vi "MGI Get Cluster Index.vi"(8 "Error In":errorcluster, 9 "Mode":T1(ring), 10 "Name":string, 11 "Cluster In":variant) -> (0 "Error Out":errorcluster, 2 "Index":i32)   [LabVIEW 2020]
doc: "This VI returns the tabbing order index of the element or subelement in <b>Cluster In</b> named <b>Name</b>. A -1 is returned if the element is not found. What <b>Index</b> means depends on <b>Mode</b>:\n\nInclude all elements and subelements: recurses all clusters and subclusters and increments for each cluster or any other data type. <b>Index</b> returns the element's order among all elements, no matter the level.\n\nFirst level only: only looks at the elements of <b>Cluster In</b>. Will not recurse on any subclusters of <b>Cluster In</b>. In this case, <b>Index</b> refers to the tabbing order of <b>Cluster In</b>.\n\nIndex in lowest level: once an element with <b>Name</b> is found, its tab order index in its owning cluster is returned in <b>Index</b>.\n\nAuthored by Robert C. Mortensen\nsupport@mooregoodideas.com\nwww.mooregoodideas.com\n\nCopyright (c) 2010, Moore Good Ideas, Inc.\n\nAll rights reserved.\n\nRedistribution and use in source and binary forms, with or without modification, are permitted provided that the following conditions are met:\n\n * Redistributions of source code must retain the above copyright notice, this list of conditions and the following disclaimer.\n * Redistributions in binary form must reproduce the above copyright notice, this list of conditions and the following disclaimer in the documentation and/or other materials provided with the distribution.\n * Neither the name of Moore Good Ideas, Inc. nor the names of its contributors may be used to endorse or promote products derived from this software without specific prior written permission.\n\nTHIS SOFTWARE IS PROVIDED BY THE COPYRIGHT HOLDERS AND CONTRIBUTORS \"AS IS\" AND ANY EXPRESS OR IMPLIED WARRANTIES, INCLUDING, BUT NOT LIMITED TO, THE IMPLIED WARRANTIES OF MERCHANTABILITY AND FITNESS FOR A PARTICULAR PURPOSE ARE DISCLAIMED. IN NO EVENT SHALL THE COPYRIGHT OWNER OR CONTRIBUTORS BE LIABLE FOR ANY DIRECT, INDIRECT, INCIDENTAL, SPECIAL, EXEMPLARY, OR CONSEQUENTIAL DAMAGES (INCLUDING, BUT NOT LIMITED TO, PROCUREMENT OF SUBSTITUTE GOODS OR SERVICES; LOSS OF USE, DATA, OR PROFITS; OR BUSINESS INTERRUPTION) HOWEVER CAUSED AND ON ANY THEORY OF LIABILITY, WHETHER IN CONTRACT, STRICT LIABILITY, OR TORT (INCLUDING NEGLIGENCE OR OTHERWISE) ARISING IN ANY WAY OUT OF THE USE OF THIS SOFTWARE, EVEN IF ADVISED OF THE POSSIBILITY OF SUCH DAMAGE."
uses:
  <vilib>/Utility/VariantDataType/VariantType.lvlib
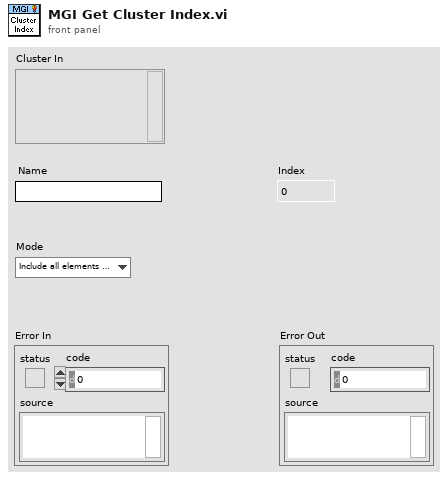
[diagram p1: front panel]
types:
  T1 = enum16{"Include all elements and subelements", "First level only", "Index in lowest level"}
  T2 = typedef "VariantType.lvlib/Type.ctl" = enum8{"Invalid Type", "Void", "I8", "I16", "I32", "I64", "U8", "U16", "U32", "U64", "Single Float", "Double Float", "Extended Float", "Single Complex", "Double Complex", "Extended Complex", "Enum U8", "Enum U16", "Enum U32", "Enum U64", "Single Float With Unit", "Double Float With Unit", "Extended Float With Unit", "Single Complex with Unit", "Double Complex with Unit", "Extended Complex with Unit", "Boolean", "String", "Path", "Picture", "Tag", "Array", "Cluster", "Variant", "LV Variant", "Waveform", "Timestamp", "Digital Waveform", "Digital Data", "ExpressData", "Refnum", "External Data", "VI", "Poly VI", "LabVIEW Class Instance", "Fixed Point"}
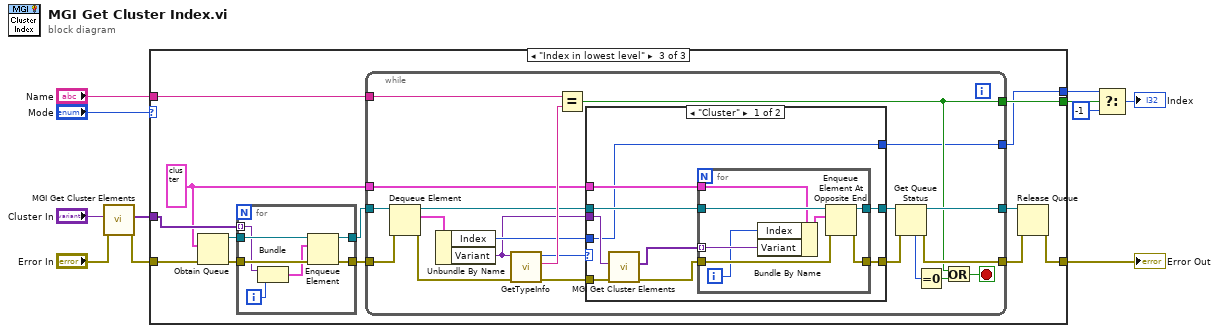
[diagram p0: block diagram]
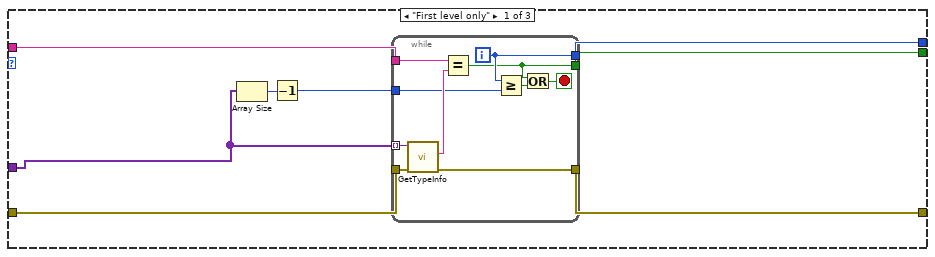
[diagram p2: hidden frame]
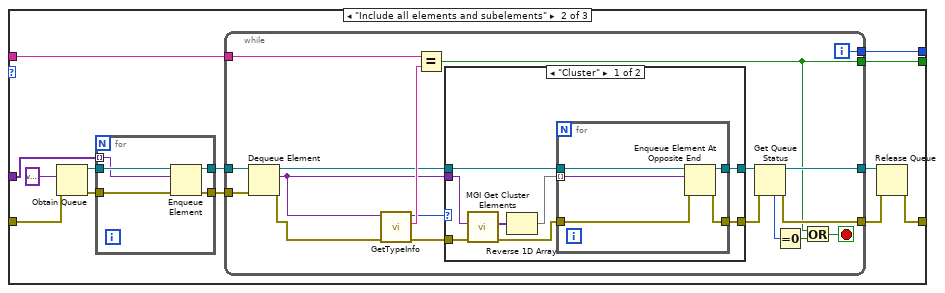
[diagram p3: hidden frame]
diagram:
  n1 = call <userlib>:"MGI Get Cluster Elements.vi"("Error In"="Error In", "Cluster"="Cluster In") -> ("Error Out"=w9:errorcluster, "Cluster Elements"=w8:variant[])  [unwired: 8 in]
  n2 = case shown="\"Index in lowest level\"" "Mode" {
    tunnel: w9 -> [w16 w42 w93]
    tunnel: w8 -> [w14 w39 w90]
    tunnel: "Name" -> [w19 w35 w87]
    tunnel: [w15 w32 w84] -> w6
    tunnel: [w18 w31 w82] -> w5
    tunnel: [w17 w30 w83] -> w2
    frame "First level only" {
      n3 = Array Size(array=w14) -> (size(s)=w13:i32)
      n4 = Decrement(x=w13) -> (x-1=w12:i32)
      n5 = while {
        tunnel: w19 -> [w28]
        tunnel: [w25] -> w15
        tunnel: [w23] -> w18
        tunnel: [w21] -> w17
        tunnel: w14 -> [w27] mode=indexing
        tunnel: w16 -> [w26]
        tunnel: w12 -> [w22]
        i -> [w23]
        stop <- w24 stop-if-true
        n6 = call <vilib>:"GetTypeInfo.vi"("error in (no error)"=w26, "Variant"=w27) -> ("error out"=w25:errorcluster, "Name"=w29:string)  [unwired: 5 in, 3 out]
        n7 = Equal?(x=w28, y=w29) -> (x = y?=w21:bool)
        n8 = Greater Or Equal?(x=w23, y=w22) -> (x >= y?=w20:bool)
        n9 = Or(x=w21, y=w20) -> (x .or. y?=w24:bool)
      }
    }
    frame "Include all elements and subelements" {
      n10 = Obtain Queue(element data type=variant, error in (no error)=w42) -> (queue out=w40:refnum<queue>, error out=w41:errorcluster)  [unwired: 3 in, 1 out]
      n11 = for {
        tunnel: w41 -> [w80]
        tunnel: w40 -> [w79]
        tunnel: w39 -> [w78] mode=indexing
        tunnel: [w77] -> w36
        tunnel: [w76] -> w37
        n12 = Enqueue Element(queue=w79, element=w78, error in (no error)=w80) -> (queue out=w76:refnum<queue>, error out=w77:errorcluster)  [unwired: 1 in, 1 out]
      }
      n13 = while {
        tunnel: w37 -> [w59]
        tunnel: w36 -> [w60]
        tunnel: w35 -> [w53]
        tunnel: [w46] -> w34
        tunnel: [w45] -> w33
        tunnel: [w44] -> w31
        tunnel: [w43] -> w30
        i -> [w44]
        stop <- w56 stop-if-true
        n14 = Dequeue Element(queue=w59, error in (no error)=w60) -> (queue out=w51:refnum<queue>, element=w47:variant, error out=w55:errorcluster)  [unwired: 1 in, 1 out]
        n15 = call <vilib>:"GetTypeInfo.vi"("error in (no error)"=w55, "Variant"=w47) -> ("error out"=w50:errorcluster, "Name"=w54:string, "Type Enum"=w52:T2)  [unwired: 5 in, 2 out]
        n16 = Equal?(x=w53, y=w54) -> (x = y?=w43:bool)
        n17 = case shown="\"Cluster\"" w52 {
          tunnel: w51 -> [w62 w75]
          tunnel: w50 -> [w67 w74]
          tunnel: w47 -> [w68 _]
          tunnel: [w65 w74] -> w49
          tunnel: [w64 w75] -> w48
          frame "Cluster" {
            n18 = call <userlib>:"MGI Get Cluster Elements.vi"("Error In"=w67, "Cluster"=w68) -> ("Error Out"=w63:errorcluster, "Cluster Elements"=w66:variant[])  [unwired: 8 in]
            n19 = Reverse 1D Array(array=w66) -> (reversed array=w61:variant[])
            n20 = for {
              tunnel: w63 -> [w73]
              tunnel: w62 -> [w72]
              tunnel: w61 -> [w71] mode=indexing
              tunnel: [w70] -> w65
              tunnel: [w69] -> w64
              n21 = Enqueue Element At Opposite End(queue=w72, element=w71, error in (no error)=w73) -> (queue out=w69:refnum<queue>, error out=w70:errorcluster)  [unwired: 1 in, 1 out]
            }
          }
          frame Default {
          }
        }
        n22 = Get Queue Status(queue=w48, error in (no error)=w49) -> (queue out=w45:refnum<queue>, error out=w46:errorcluster, # elements in queue=w58:i32)  [unwired: 1 in, 5 out]
        n23 = Equal To 0?(x=w58) -> (x = 0?=w57:bool)
        n24 = Or(x=w43, y=w57) -> (x .or. y?=w56:bool)
      }
      n25 = Release Queue(queue=w33, error in (no error)=w34) -> (error out=w32:errorcluster)  [unwired: 1 in, 2 out]
    }
    frame "Index in lowest level" {
      w81 = cluster{"Variant":variant, "Index":i32} {"Variant"=variant, "Index"=0} ("cluster")
      n26 = Obtain Queue(element data type=w81, error in (no error)=w93) -> (queue out=w91:refnum<queue>, error out=w92:errorcluster)  [unwired: 3 in, 1 out]
      n27 = for {
        tunnel: w92 -> [w141]
        tunnel: w91 -> [w140]
        tunnel: w90 -> [w139] mode=indexing
        tunnel: [w138] -> w88
        tunnel: [w137] -> w89
        i -> [w135]
        n28 = Bundle("Variant"=w139, w135) -> (w136:cluster{"Variant":variant, i32})  [unwired: 1 in]
        n29 = Enqueue Element(queue=w140, element=w136, error in (no error)=w141) -> (queue out=w137:refnum<queue>, error out=w138:errorcluster)  [unwired: 1 in, 1 out]
      }
      n30 = while {
        tunnel: w89 -> [w113]
        tunnel: w88 -> [w114]
        tunnel: w87 -> [w107]
        tunnel: [w101] -> w86
        tunnel: [w100] -> w85
        tunnel: [w99] -> w83
        tunnel: w81 -> [w96]
        tunnel: [w98] -> w82
        stop <- w110 stop-if-true
        n31 = Dequeue Element(queue=w113, error in (no error)=w114) -> (queue out=w105:refnum<queue>, element=w97:cluster{"Variant":variant, "Index":i32}, error out=w109:errorcluster)  [unwired: 1 in, 1 out]
        n32 = Unbundle By Name(w97) -> ("Index"=w95:i32, "Variant"=w94:variant)
        n33 = call <vilib>:"GetTypeInfo.vi"("error in (no error)"=w109, "Variant"=w94) -> ("error out"=w104:errorcluster, "Name"=w108:string, "Type Enum"=w106:T2)  [unwired: 5 in, 2 out]
        n34 = Equal?(x=w107, y=w108) -> (x = y?=w99:bool)
        n35 = case shown="\"Cluster\"" w106 {
          tunnel: w105 -> [w118 w134]
          tunnel: w104 -> [w122 w133]
          tunnel: w94 -> [w123 _]
          tunnel: [w121 w133] -> w103
          tunnel: [w120 w134] -> w102
          tunnel: [w116 w132] -> w98
          tunnel: w96 -> [w117 _]
          tunnel: w95 -> [w116 w132]
          frame "Cluster" {
            n36 = call <userlib>:"MGI Get Cluster Elements.vi"("Error In"=w122, "Cluster"=w123) -> ("Error Out"=w119:errorcluster, "Cluster Elements"=w115:variant[])  [unwired: 8 in]
            n37 = for {
              tunnel: w119 -> [w131]
              tunnel: w118 -> [w130]
              tunnel: w115 -> [w129] mode=indexing
              tunnel: [w128] -> w121
              tunnel: [w127] -> w120
              tunnel: w117 -> [w126]
              i -> [w124]
              n38 = Bundle By Name(cluster=w126, "Index"=w124, "Variant"=w129) -> (w125:cluster{"Variant":variant, "Index":i32})
              n39 = Enqueue Element At Opposite End(queue=w130, element=w125, error in (no error)=w131) -> (queue out=w127:refnum<queue>, error out=w128:errorcluster)  [unwired: 1 in, 1 out]
            }
          }
          frame Default {
          }
        }
        n40 = Get Queue Status(queue=w102, error in (no error)=w103) -> (queue out=w100:refnum<queue>, error out=w101:errorcluster, # elements in queue=w112:i32)  [unwired: 1 in, 5 out]
        n41 = Equal To 0?(x=w112) -> (x = 0?=w111:bool)
        n42 = Or(x=w99, y=w111) -> (x .or. y?=w110:bool)
      }
      n43 = Release Queue(queue=w85, error in (no error)=w86) -> (error out=w84:errorcluster)  [unwired: 1 in, 2 out]
    }
  }
  "Error Out" <- w6
  n44 = Select(t=w5, s=w2, f=-1) -> (s? t:f=→"Index":i32)
